vi "Process.vi"(8 "error in":errorcluster, 11 "Logger.syslog":refnum<class "Logger.syslog.lvclass">) -> (0 "error out":errorcluster, 3 "Logger.syslog out":refnum<class "Logger.syslog.lvclass">)   [LabVIEW 2019, in "Logger.syslog.lvlib" / "Logger.syslog.lvclass"]
doc: "---------------------------------------------------------------\nJKI State Machine Objects™\nhttp://jki.net/state-machine-objects/\nCopyright (C) 2005-2015, JKI <info@jki.net>\nALL RIGHTS RESERVED"
uses:
  Logger.syslog.lvclass
  <vilib>/NI/syslog/_subVIs/TypeDefs/syslog_message_cluster.ctl
  <vilib>/NI/syslog/_subVIs/TypeDefs/syslog_facility_codes.ctl
  <vilib>/NI/syslog/_subVIs/TypeDefs/syslog_severity_codes.ctl
  Typedefs/PrivateEvents--Logger.syslog.syslog message.ctl
  Logger.syslog.lvclass/Logger.syslog.ctl
  <userlib>/LevyLab/Logger/Logger/Logger.lvclass
  <vilib>/JKI/JKI SMO/smo.lvlibp/SMO/SMO.lvclass
  C:/Program Files (x86)/National Instruments/LabVIEW 2019/user.lib/LevyLab/Logger/Logger/Logger.lvclass
  C:/Program Files (x86)/National Instruments/LabVIEW 2019/vi.lib/JKI/JKI SMO/smo.lvlibp/SMO/SMO.lvclass
  <userlib>/LevyLab/Debug/Debug.lvlib
panel:
  # "For instructions on how to use the JKI State Machine Objects, examples and video tutorials, visit:\nhttp://jki.net/state-machine-objects/\n\nJKI State Machine Objects™\nhttp://jki.net/state-machine-objects/\nCopyright (C) 2005-2015, JKI <info@jki.net>\nALL RIGHTS RESERVED"
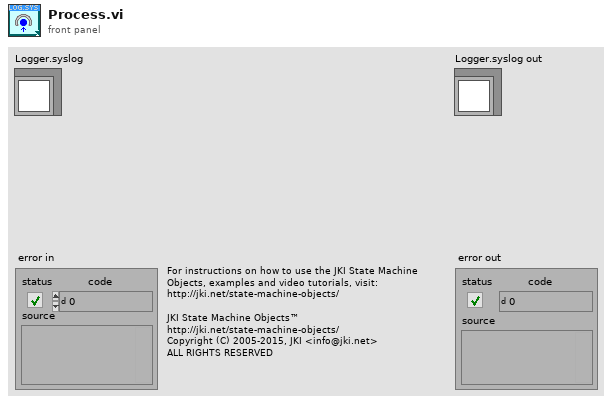
[diagram p1: front panel]
types:
  T1 = enum32{"invalid app kind", "Development System", "Run Time System", "Student Edition", "Embedded LabVIEW", "Evaluation", "Custom"}
  T2 = enum32{"Invalid", "Standard", "Closed", "Hidden", "Minimized", "Maximized"}
  T3 = enum16{"open", "replace", "create", "open or create", "replace or create", "replace or create with confirmation"}
  T4 = typedef "Logger.syslog.lvlib/Logger.syslog.lvclass/PrivateEvents--Logger.syslog.syslog message.ctl" = string
  T5 = typedef "syslog_message_cluster.ctl" = cluster{"Facility Code":T6, "Severity Code":T7, "Time Stamp":timestamp, "Hostname":string, "Message Tag":string, "Message Content":string}
  T6 = typedef "syslog_facility_codes.ctl" = enum16{"kernel", "user", "mail", "system daemons", "security/authorization", "syslogd", "line printer", "network news", "uucp", "clock daemon", "security/authorization (alternate)", "FTP daemon", "NTP subsystem", "log audit", "log alert", "clock daemon (alternate)", "local use 0", "local use 1", "local use 2", "local use 3", "local use 4", "local use 5", "local use 6", "local use 7"}
  T7 = typedef "syslog_severity_codes.ctl" = enum16{"emergency", "alert", "critical", "error", "warning", "notice", "info", "debug"}
  T8 = cluster{"Core":cluster{"Current VI Reference":refnum<vi>, "Close Panel on Exit?":bool, "Last Error":cluster{"error":errorcluster, "previous state":string, "remaining states":string}, "Shutdown?":bool}, "SelfRef":refnum<class "Logger.syslog.lvclass">, "collector port (514)":u16, "Syslog Collector Ref":refnum<k16>, "syslog message":T4, "Syslog Message":T5, "path":path}
  T9 = cluster{"Current VI Reference":refnum<vi>, "Close Panel on Exit?":bool, "Last Error":cluster{"error":errorcluster, "previous state":string, "remaining states":string}, "Shutdown?":bool}
  T10 = typedef "Debug.lvlib/Attribute.Debug.lvclass/DebugBehavior.ctl" = enum16{"Normal", "Debug"}
  T11 = typedef "smo.lvlibp/SMO.lvclass/Protected Events.ctl" = cluster{"StopProcesses":refnum<user-event>, "AbortProcesses":refnum<user-event>, "Config Changed":refnum<user-event>, "Dependency":refnum<user-event>}
  T12 = typedef "Logger.syslog.lvlib/Logger.syslog.lvclass/PrivateEvents--Cluster.ctl" = cluster{"syslog message":refnum<user-event>}
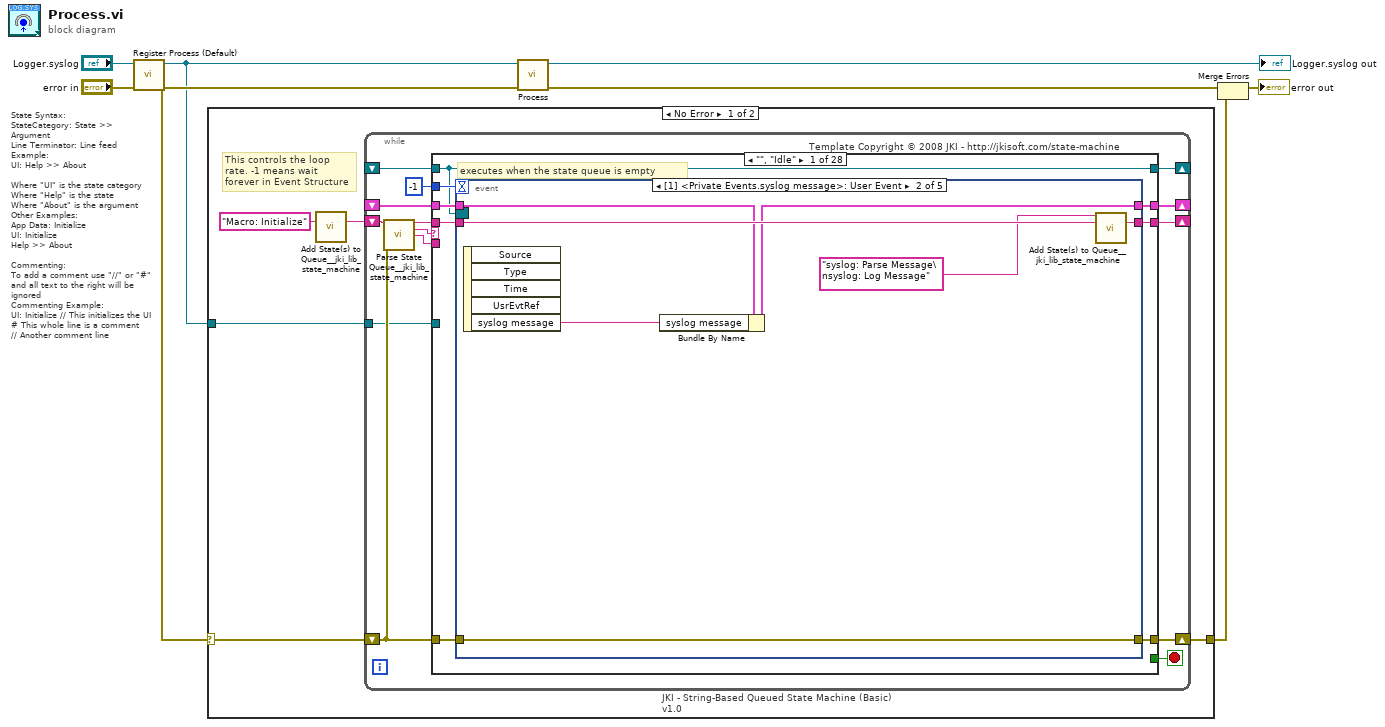
[diagram p0: block diagram]
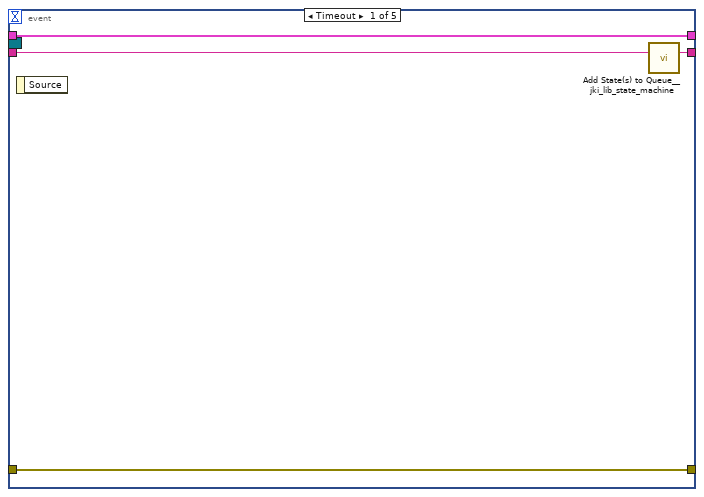
[diagram p2: hidden frame]
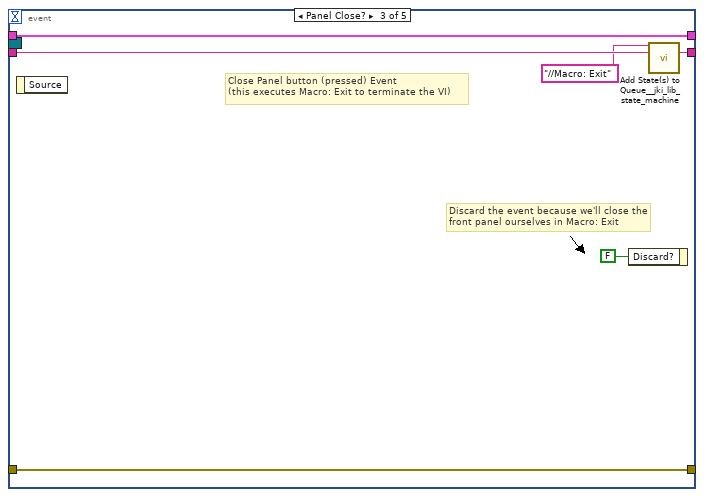
[diagram p3: hidden frame]
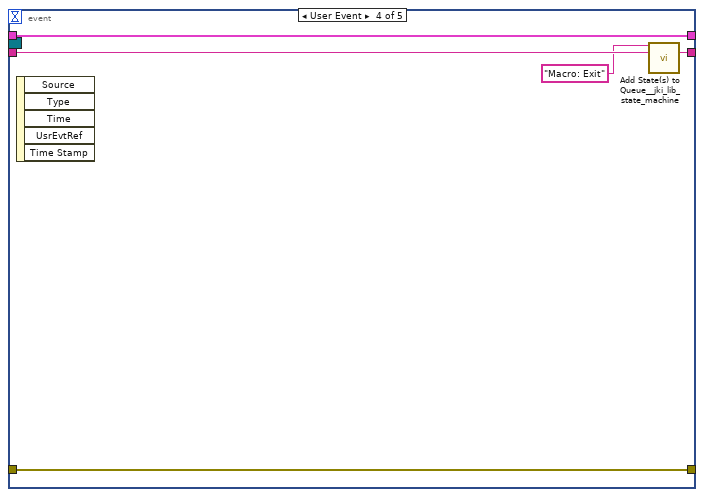
[diagram p4: hidden frame]
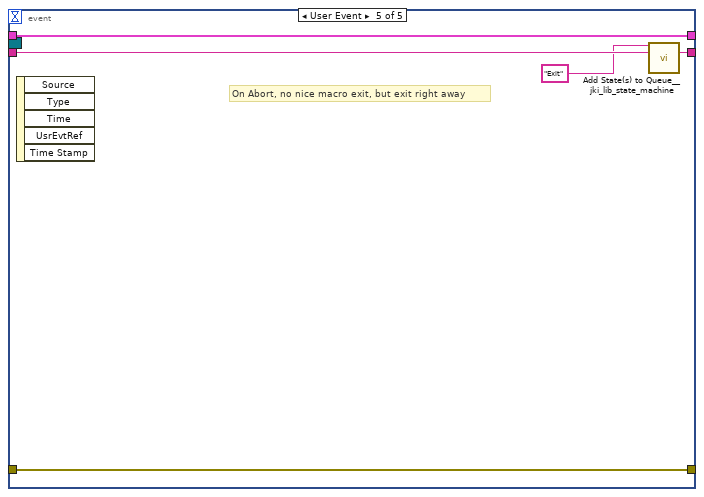
[diagram p5: hidden frame]
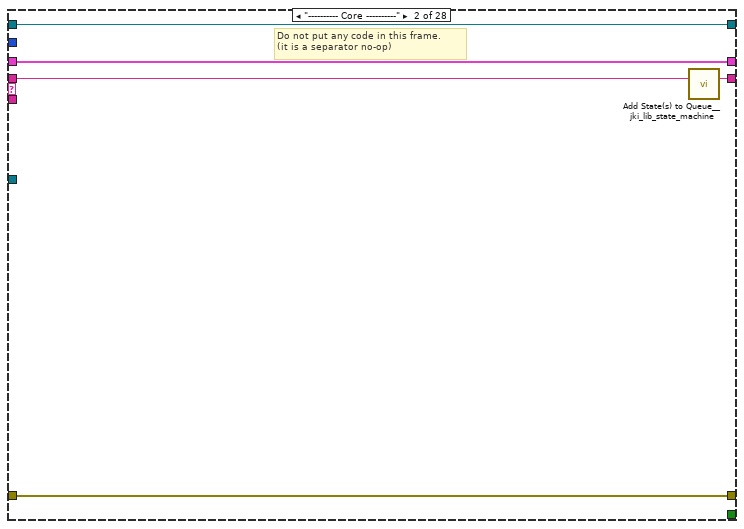
[diagram p6: hidden frame]
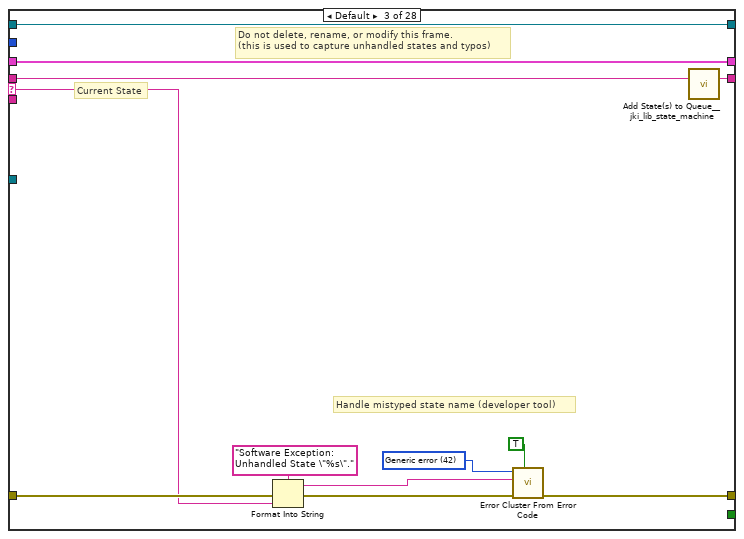
[diagram p7: hidden frame]
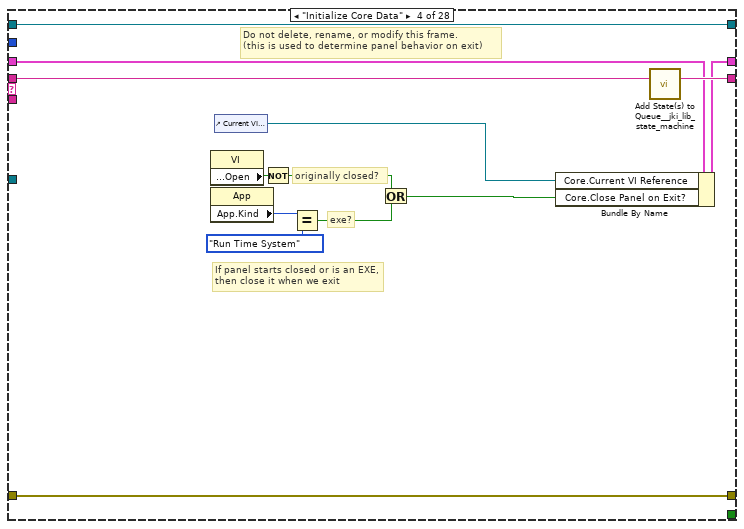
[diagram p8: hidden frame]
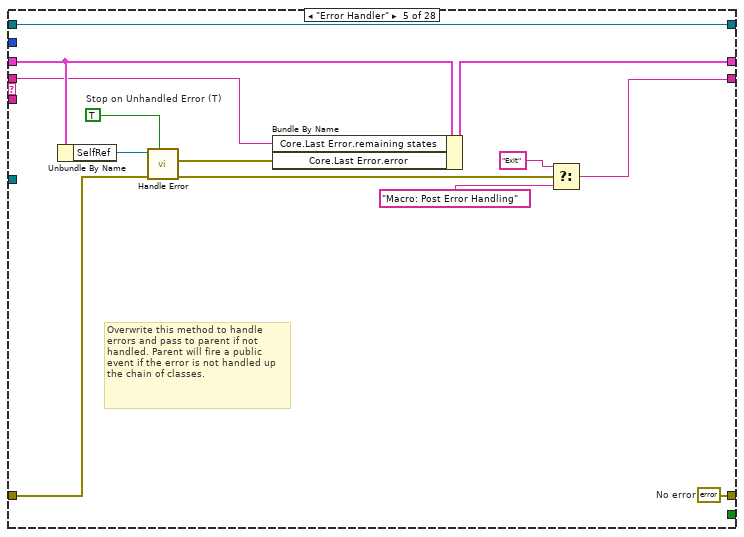
[diagram p9: hidden frame]
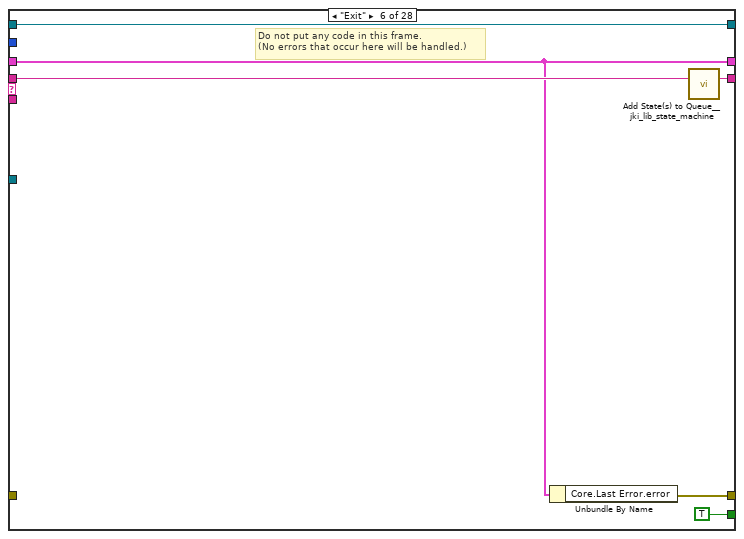
[diagram p10: hidden frame]
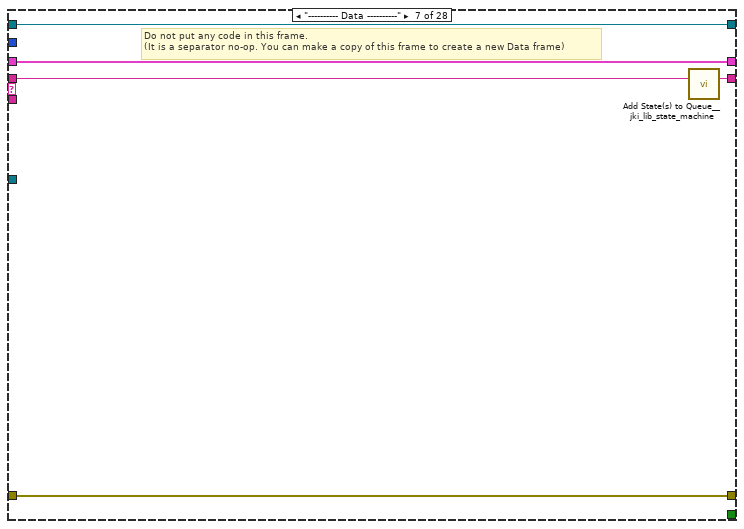
[diagram p11: hidden frame]
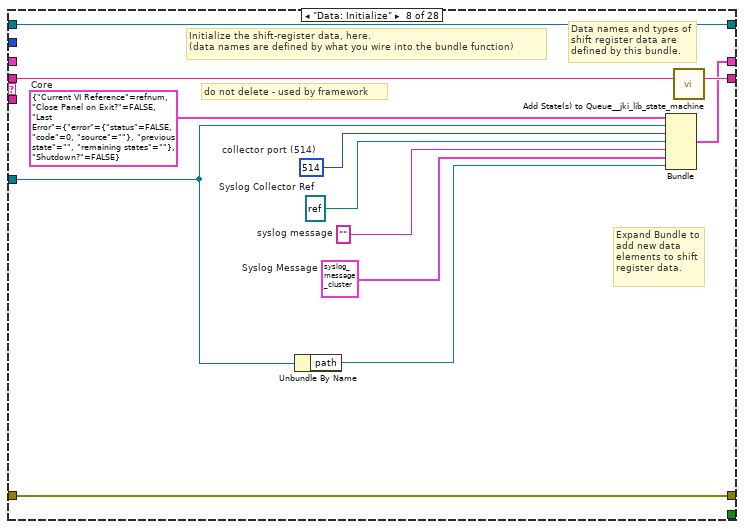
[diagram p12: hidden frame]
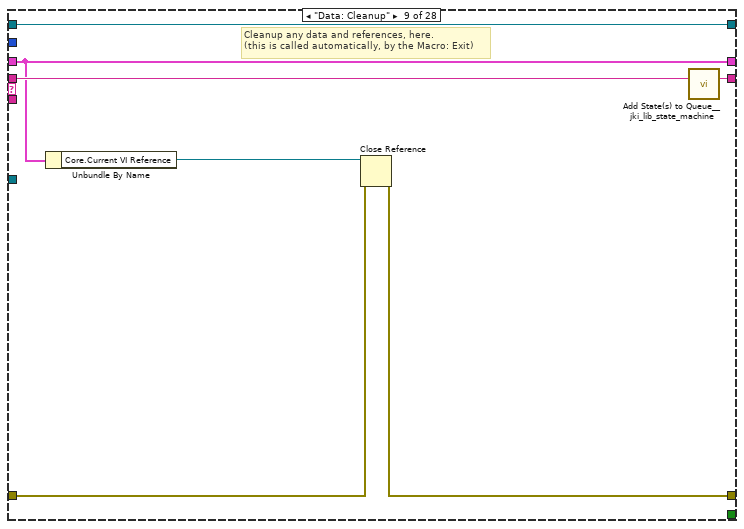
[diagram p13: hidden frame]
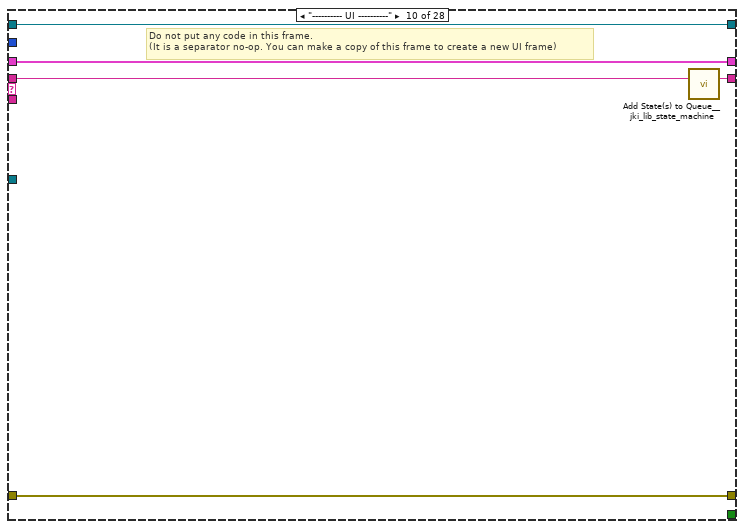
[diagram p14: hidden frame]
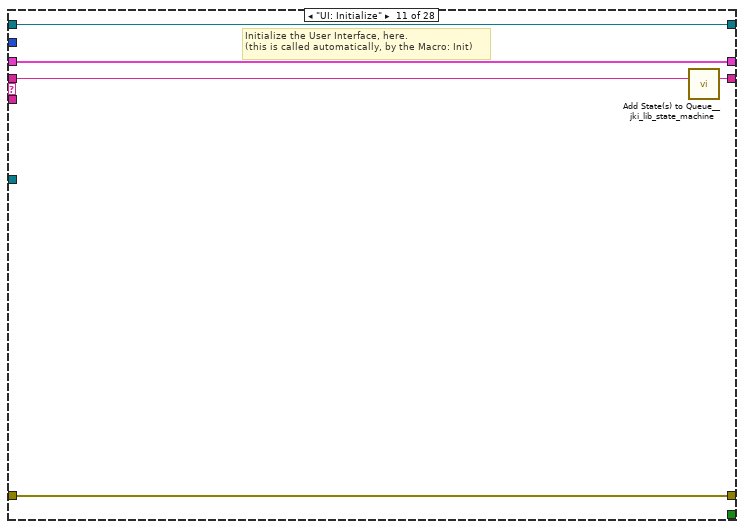
[diagram p15: hidden frame]
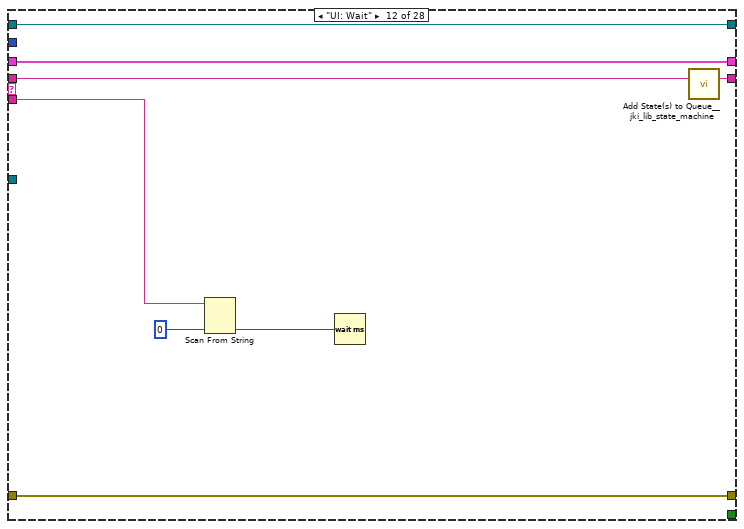
[diagram p16: hidden frame]
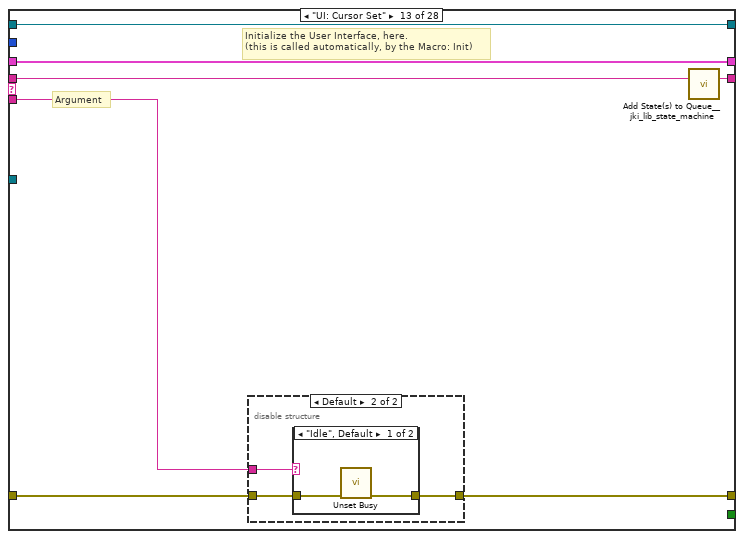
[diagram p17: hidden frame]
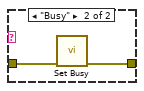
[diagram p19: hidden frame]
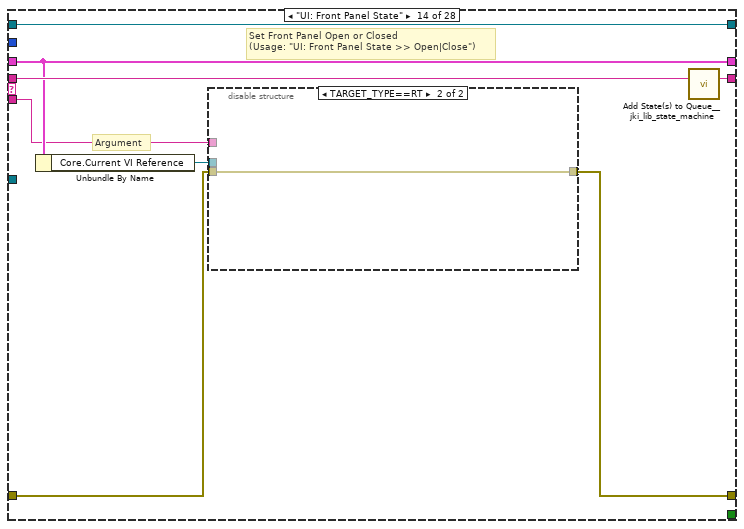
[diagram p20: hidden frame]
diagram:
  # "State Syntax:\nStateCategory: State >> Argument\nLine Terminator: Line feed\nExample:\nUI: Help >> About\n\nWhere \"UI\" is the state category\nWhere \"Help\" is the state\nWhere \"About\" is the argument\nOther Examples:\nApp Data: Initialize\nUI: Initialize\nHelp >> About\n\nCommenting:\nTo add a comment use \"//\" or \"#\" and all text to the right will be ignored\nCommenting Example:\nUI: Initialize // This initializes the UI\n# This whole line is a comment\n// Another comment line"
  n1 = call <vilib>:"Register Process (Default).vi"("error in (no error)"="error in", "SMO"="Logger.syslog") -> ("error out"=w5:errorcluster, "SelfRef"=w4:refnum<class "Logger.syslog.lvclass">)  [unwired: 8 in]
  n2 = case shown="No Error" w5 {
    selector: w5 -> [w10 w362]
    tunnel: w4 -> [w11 _]
    tunnel: [w9 w362] -> w1
    frame No Error {
      # "This controls the loop rate. -1 means wait forever in Event Structure"
      n3 = call <vilib>:"Add State(s) to Queue__jki_lib_state_machine.vi"("State(s) in (\"\")"="Macro: Initialize") -> ("States Out"=w13:string)  [unwired: 14 in]
      n4 = while "JKI - String-Based Queued State Machine (Basic) v1.0" {
        shift-right: [w20] -> _
        shift-left: _ -> [w19]
        shift-right: [w23] -> w9
        shift-left: w10 -> [w17]
        shift-right: [w22] -> _
        shift-left: w13 -> [w24]
        tunnel: w11 -> [w16]
        shift-right: [w15] -> _
        shift-left: _ -> [w14]
        stop <- w21 stop-if-true
        # "Template Copyright © 2008 JKI - http://jkisoft.com/state-machine"
        n5 = call <vilib>:"Parse State Queue__jki_lib_state_machine.vi"("State Queue"=w24, "Error In (no error)"=w17) -> ("Remaining States"=w26:string, "Current State"=w27:string, "Arguments"=w25:string)  [unwired: 11 in]
        n6 = case shown="\"\", \"Idle\"" w27 {
          selector: w27 -> [_ _ w69 _ _ _ _ _ _ _ _ _ _ _ _ _ _ _ _ _ _ _ _ _ _ _ _ _]
          tunnel: w26 -> [w35 w67 w73 w92 w93 w111 w116 w128 w135 w140 w145 w153 w160 w176 w208 w217 w232 w249 w269 w274 w285 w290 w303 w309 w314 w323 w331 w340]
          tunnel: w25 -> [_ _ _ _ _ _ _ _ _ _ _ w146 w154 w170 _ _ _ _ _ _ _ _ _ _ _ _ _ _]
          tunnel: w19 -> [w33 w64 w71 w83 w101 w107 w113 _ w130 w137 w143 w150 w158 w172 w205 w213 w221 w238 w255 w271 w282 w287 w301 w307 w312 w320 w325 w337]
          tunnel: [w32 w65 w75 w89 w102 w106 w114 w117 w131 w138 w142 w151 w155 w173 w206 w215 w219 w247 w267 w272 w276 w288 w296 w305 w310 w315 w328 w334] -> w23
          tunnel: w17 -> [w31 w65 w74 w89 w103 _ w114 w117 w132 w138 w142 w151 w156 w174 w206 w215 w218 w247 w267 w272 w277 w288 w297 w305 w310 w316 w328 w335]
          tunnel: [w34 w66 w72 w91 w95 w110 w115 w127 w134 w139 w144 w152 w159 w175 w207 w216 w231 w248 w268 w273 w284 w289 w302 w308 w313 w322 w330 w339] -> w22
          tunnel: [_ _ _ _ _ TRUE _ _ _ _ _ _ _ _ _ _ _ _ _ _ _ _ _ _ _ _ _ _] -> w21
          tunnel: [w30 w64 w71 w90 w100 w107 w113 w126 w130 w137 w143 w150 w158 w172 w205 w213 w222 w240 w256 w271 w282 w287 w301 w307 w312 w319 w326 w337] -> w20
          tunnel: -1 ("Timeout") -> [w29 _ _ _ _ _ _ _ _ _ _ _ _ _ _ _ _ _ _ _ _ _ _ _ _ _ _ _]
          tunnel: w16 -> [_ _ _ _ _ _ _ w118 _ _ _ _ _ _ _ _ _ _ _ _ _ _ _ _ _ _ _ _]
          tunnel: [w28 w63 w68 w80 w105 w108 w112 w125 w129 w136 w141 w149 w157 w169 w204 w214 w230 w246 w261 w270 w283 w286 w300 w306 w311 w321 w329 w338] -> w15
          tunnel: w14 -> [w28 w63 w68 w80 w105 w108 w112 w125 w129 w136 w141 w149 w157 w169 w204 w214 w230 w246 w261 w270 w283 w286 _ w306 w311 w321 w329 w338]
          frame "", "Idle" {
            # "executes when the state queue is empty"
            n7 = event shown="[1] <Private Events.syslog message>: User Event" {
              selector: w28 -> [_ _ _ _ _]
              dyn-events: _ -> [_ _ _ _ _]
              timeout: w29 -> [_ _ _ _ _]
              tunnel: w35 -> [w39 w46 w52 w57 w62]
              tunnel: [w38 w45 w51 w56 w61] -> w34
              tunnel: w33 -> [w37 w43 w49 w54 w59]
              tunnel: [w36 w44 w50 w55 w60] -> w32
              tunnel: w31 -> [w36 w44 w50 w55 w60]
              tunnel: [w37 w42 w49 w54 w59] -> w30
              event Timeout {
                n8 = event-data() -> ()  [unwired: 1 in, 1 out]
                n9 = call <vilib>:"Add State(s) to Queue__jki_lib_state_machine.vi"("State(s) in (\"\")"=w39) -> ("States Out"=w38:string)  [unwired: 14 in]
              }
              event User Event {
                n10 = event-data() -> ("syslog message"=w41:T4)  [unwired: 1 in, 4 out]
                n11 = Bundle By Name(cluster=w43, "syslog message"=w41) -> (w42:T8)
                n12 = call <vilib>:"Add State(s) to Queue__jki_lib_state_machine.vi"("State(s) in Front (\"\")"="syslog: Parse Message\nsyslog: Log Message" ("State(s) in Front (\"\")"), "State(s) in (\"\")"=w46) -> ("States Out"=w45:string)  [unwired: 13 in]
              }
              event Panel Close? {
                # "Discard the event because we'll close the front panel ourselves in Macro: Exit"
                # "Close Panel button (pressed) Event\n(this executes Macro: Exit to terminate the VI)"
                n13 = event-data() -> ()  [unwired: 1 in, 1 out]
                n14 = event-data("Discard?"=FALSE) -> ()  [unwired: 1 in, 1 out]
                n15 = call <vilib>:"Add State(s) to Queue__jki_lib_state_machine.vi"("State(s) in Front (\"\")"="//Macro: Exit", "State(s) in (\"\")"=w52) -> ("States Out"=w51:string)  [unwired: 13 in]
              }
              event User Event {
                n16 = event-data() -> ()  [unwired: 1 in, 5 out]
                n17 = call <vilib>:"Add State(s) to Queue__jki_lib_state_machine.vi"("State(s) in Front (\"\")"="Macro: Exit", "State(s) in (\"\")"=w57) -> ("States Out"=w56:string)  [unwired: 13 in]
              }
              event User Event {
                # "On Abort, no nice macro exit, but exit right away"
                n18 = event-data() -> ()  [unwired: 1 in, 5 out]
                n19 = call <vilib>:"Add State(s) to Queue__jki_lib_state_machine.vi"("State(s) in Front (\"\")"="Exit", "State(s) in (\"\")"=w62) -> ("States Out"=w61:string)  [unwired: 13 in]
              }
            }
          }
          frame "---------- Core ----------" {
            # "Do not put any code in this frame.\n(it is a separator no-op)"
            n20 = call <vilib>:"Add State(s) to Queue__jki_lib_state_machine.vi"("State(s) in (\"\")"=w67) -> ("States Out"=w66:string)  [unwired: 14 in]
          }
          frame Default {
            w78 = 42 items=["No error", "Argument error", "Memory is full", "Out of zone", "End of file", "File already open", "Generic file I/O error", "File not found", "File permission error", "Disk is full", "Duplicate path", "Too many files open", "System feature not enabled", "Resource file not found", "Cannot add resource", "Resource not found", "Image not found", "Image memory error", "Pen does not exist", "Config type invalid", "Config token not found", "Config parse error", "Config memory error", "Bad external code format", "Bad external code offset", "External code not present", "Null window", "Destroy window error", "Null menu", "Print aborted", "Bad print record", "Print driver error", "Windows error during printing", "Memory error during printing", "Print dialog error", "Generic print error", "Invalid device refnum", "Device not found", "Device parameter error", "Device unit error", "Cannot open device", "Device call aborted", "Generic error", "Cancelled by user", "Object ID too low", "Object ID too high", "Object not in heap", "Unknown heap", "Unknown object (invalid DefProc)", "Unknown object (DefProc not in table)", "Message out of range", "Invalid (null) method", "Unknown message", "Manager call not supported", "Bad address", "Network operation in progress", "Network operation timed out", "Connection is busy", "Network attribute not supported", "Network error", "Address in use", "System out of memory", "Connection aborted", "Connection refused", "Not connected", "Already connected", "Connection closed", "Initialization error (interapplication manager)", "Bad occurrence", "Wait on unbound occurrence handler", "Occurrence queue overflow", "Datalog type conflict", "Unused", "Unrecognized type (interapplication manager)", "Memory corrupt", "Failed to make temporary DLL", "Old CIN version", "Drag socket not found", "Failed to load drop-object", "Failed to register OLE object", "Failed to release OLE object", "Format specifier type mismatch", "Unknown format specifier", "Too few format specifiers", "Too many format specifiers", "Scan failed", "Newer CIN version", "Error converting to variant", "Runtime menu error", "Password tampered", "Variant attribute not found", "Incompatible variant data type", "Event data is not available", "Event Store is not present", "Occurrence is not found", "Event Queue is not created", "Event info is not available", "Refnum passed is NULL", "Error retrieving Class GUID", "Error retrieving CoClass GUID", "Error retrieving TypeLib GUID.", "Bad built application magic bytes.", "Specific driver is different from the specific driver associated with the Logical Name.", "There is no session opened to the class driver.", "Max Error", "MAX - Error with config objects", "MAX - Error loading configuration", "MAX - Group not supported"]
            # "Current State"
            # "Do not delete, rename, or modify this frame.\n(this is used to capture unhandled states and typos)"
            # "Handle mistyped state name (developer tool)"
            n21 = Format Into String(format string="Software Exception: Unhandled State \"%s\"." ("message"), error in=w74, w69) -> (resulting string=w77:string, error out=w76:errorcluster)  [unwired: 1 in]
            n22 = call <vilib>:"Error Cluster From Error Code.vi"("show call chain? (False)"=TRUE, "error in (no error)"=w76, "error message (\"\")"=w77, "error code (0)"=w78) -> ("error out"=w75:errorcluster)  [unwired: 5 in]
            n23 = call <vilib>:"Add State(s) to Queue__jki_lib_state_machine.vi"("State(s) in (\"\")"=w73) -> ("States Out"=w72:string)  [unwired: 14 in]
          }
          frame "Initialize Core Data" {
            # "Do not delete, rename, or modify this frame.\n(this is used to determine panel behavior on exit)"
            # "originally closed?"
            # "exe?"
            # "If panel starts closed or is an EXE, then close it when we exit"
            n24 = property class="VI"() -> ("Front Panel.Open"=w88:bool)  [unwired: 2 in, 2 out]
            n25 = property class="App"() -> ("App.Kind"=w87:T1)  [unwired: 2 in, 2 out]
            n26 = control-ref of="Current VI Reference"() -> (w81:refnum<vi>)
            n27 = Not(x=w88) -> (.not. x?=w85:bool)
            n28 = Equal?(x=w87, y=T1."Run Time System" ("Application:Kind")) -> (x = y?=w84:bool)
            n29 = Or(x=w85, y=w84) -> (x .or. y?=w82:bool)
            n30 = Bundle By Name(cluster=w83, "Core.Current VI Reference"=w81, "Core.Close Panel on Exit?"=w82) -> (w90:T8)
            n31 = call <vilib>:"Add State(s) to Queue__jki_lib_state_machine.vi"("State(s) in (\"\")"=w92) -> ("States Out"=w91:string)  [unwired: 14 in]
          }
          frame "Error Handler" {
            w96 = TRUE  # Stop on Unhandled Error (T)
            w102 = errorcluster {"status"=FALSE, "code"=0, "source"=""}  # No error
            # "Overwrite this method to handle errors and pass to parent if not handled. Parent will fire a public event if the error is not handled up the chain of classes."
            n32 = Unbundle By Name(w101) -> ("SelfRef"=w104:refnum<class "Logger.syslog.lvclass">)
            n33 = call-dynamic "Handle Error.vi"("Stop on Unhandled Error (T)"=w96, "error in"=w103, "SMO"=w104) -> ("handling error"=w97:errorcluster, "Unhandled error"=w99:errorcluster)  [unwired: 6 in, 1 out]
            n34 = Bundle By Name(cluster=w101, "Core.Last Error.remaining states"=w93, "Core.Last Error.error"=w99) -> (w100:T8)
            n35 = Select(t="Exit", s=w97, f="Macro: Post Error Handling") -> (s? t:f=w95:string)
          }
          frame "Exit" {
            # "Do not put any code in this frame.\n(No errors that occur here will be handled.)"
            n36 = Unbundle By Name(w107) -> ("Core.Last Error.error"=w106:errorcluster)
            n37 = call <vilib>:"Add State(s) to Queue__jki_lib_state_machine.vi"("State(s) in (\"\")"=w111) -> ("States Out"=w110:string)  [unwired: 14 in]
          }
          frame "---------- Data ----------" {
            # "Do not put any code in this frame.\n(It is a separator no-op. You can make a copy of this frame to create a new Data frame)"
            n38 = call <vilib>:"Add State(s) to Queue__jki_lib_state_machine.vi"("State(s) in (\"\")"=w116) -> ("States Out"=w115:string)  [unwired: 14 in]
          }
          frame "Data: Initialize" {
            w121 = T4 ""  # syslog message
            w120 = T5 {"Facility Code"=enum."kernel", "Severity Code"=enum."emergency", "Time Stamp"=timestamp(0 s since 1904-01-01), "Hostname"="", "Message Tag"="", "Message Content"=""}  # Syslog Message
            w122 = refnum<k16> refnum  # Syslog Collector Ref
            w123 = u16 514  # collector port (514)
            w124 = T9 {"Current VI Reference"=refnum, "Close Panel on Exit?"=FALSE, "Last Error"={"error"={"status"=FALSE, "code"=0, "source"=""}, "previous state"="", "remaining states"=""}, "Shutdown?"=FALSE}  # Core
            # "do not delete - used by framework"
            # "Expand Bundle to add new data elements to shift register data."
            # "Data names and types of shift register data are defined by this bundle."
            # "Initialize the shift-register data, here.\n(data names are defined by what you wire into the bundle function)"
            n39 = Unbundle By Name(w118) -> ("path"=w119:path)
            n40 = Bundle("Core"=w124, "SelfRef"=w118, "collector port (514)"=w123, "Syslog Collector Ref"=w122, "syslog message"=w121, "Syslog Message"=w120, "path"=w119) -> (w126:T8)  [unwired: 1 in]
            n41 = call <vilib>:"Add State(s) to Queue__jki_lib_state_machine.vi"("State(s) in (\"\")"=w128) -> ("States Out"=w127:string)  [unwired: 14 in]
          }
          frame "Data: Cleanup" {
            # "Cleanup any data and references, here.\n(this is called automatically, by the Macro: Exit)"
            n42 = Unbundle By Name(w130) -> ("Core.Current VI Reference"=w133:refnum<vi>)
            n43 = Close Reference(reference=w133, error in (no error)=w132) -> (error out=w131:errorcluster)
            n44 = call <vilib>:"Add State(s) to Queue__jki_lib_state_machine.vi"("State(s) in (\"\")"=w135) -> ("States Out"=w134:string)  [unwired: 14 in]
          }
          frame "---------- UI ----------" {
            # "Do not put any code in this frame.\n(It is a separator no-op. You can make a copy of this frame to create a new UI frame)"
            n45 = call <vilib>:"Add State(s) to Queue__jki_lib_state_machine.vi"("State(s) in (\"\")"=w140) -> ("States Out"=w139:string)  [unwired: 14 in]
          }
          frame "UI: Initialize" {
            # "Initialize the User Interface, here.\n(this is called automatically, by the Macro: Init)"
            n46 = call <vilib>:"Add State(s) to Queue__jki_lib_state_machine.vi"("State(s) in (\"\")"=w145) -> ("States Out"=w144:string)  [unwired: 14 in]
          }
          frame "UI: Wait" {
            n47 = Scan From String(input string=w146, default 1=u32 0) -> (output 1=w147:u32)  [unwired: 3 in, 3 out]
            n48 = Wait (ms)(milliseconds to wait=w147) -> ()  [unwired: 1 out]
            n49 = call <vilib>:"Add State(s) to Queue__jki_lib_state_machine.vi"("State(s) in (\"\")"=w153) -> ("States Out"=w152:string)  [unwired: 14 in]
          }
          frame "UI: Cursor Set" {
            # "Argument"
            # "Initialize the User Interface, here.\n(this is called automatically, by the Macro: Init)"
            n50 = disable-structure shown="Default" {
              disable-tunnel: w156 -> [w161 w164]
              disable-tunnel: [w161 w163] -> w155
              disable-tunnel: w154 -> [_ w162]
              frame condition #0 {
              }
              frame condition #1 (active) {
                n51 = case shown="\"Idle\", Default" w162 {
                  tunnel: w164 -> [w166 w168]
                  tunnel: [w165 w167] -> w163
                  frame "Idle", Default {
                    n52 = call <vilib>:"Unset Busy.vi"("error in (no error)"=w166) -> ("error out"=w165:errorcluster)  [unwired: 10 in]
                  }
                  frame "Busy" {
                    n53 = call <vilib>:"Set Busy.vi"("error in (no error)"=w168) -> ("error out"=w167:errorcluster)  [unwired: 9 in, 1 out]
                  }
                }
              }
            }
            n54 = call <vilib>:"Add State(s) to Queue__jki_lib_state_machine.vi"("State(s) in (\"\")"=w160) -> ("States Out"=w159:string)  [unwired: 14 in]
          }
          frame "UI: Front Panel State" {
            # "Argument"
            # "Set Front Panel Open or Closed\n(Usage: \"UI: Front Panel State >> Open|Close\")"
            n55 = Unbundle By Name(w172) -> ("Core.Current VI Reference"=w171:refnum<vi>)
            n56 = disable-structure shown="TARGET_TYPE==RT" {
              disable-tunnel: w174 -> [w180 w203]
              disable-tunnel: [w179 w203] -> w173
              disable-tunnel: w171 -> [w178 _]
              disable-tunnel: w170 -> [w177 _]
              frame condition #0 (active) {
                n57 = case shown="\"Close\"" w177 {
                  tunnel: w180 -> [w184 w197]
                  tunnel: [w186 w198] -> w179
                  tunnel: w178 -> [w185 w195]
                  frame "Open", Default {
                    n58 = property class="VI"(reference=w185, error in=w184) -> (reference out=w182:refnum<vi>, error out=w183:errorcluster, "FP.State"=w181:T2)
                    n59 = case shown="\"Closed\"" w181 {
                      tunnel: [w189 w192] -> w186
                      tunnel: w183 -> [w188 w192]
                      tunnel: w182 -> [w187 _]
                      frame "Closed" {
                        n60 = invoke class="VI" method="FP.Open"(reference=w187, error in=w188, "Activate"=TRUE, "State"=T2."Standard") -> (error out=w189:errorcluster)  [unwired: 1 in, 4 out]
                      }
                      frame Default {
                      }
                    }
                  }
                  frame "Close" {
                    n61 = property class="VI"(reference=w195, error in=w197) -> (reference out=w194:refnum<vi>, error out=w196:errorcluster, "FP.State"=w193:T2)
                    n62 = case shown="Default" w193 {
                      tunnel: [w199 w202] -> w198
                      tunnel: w196 -> [w199 w201]
                      tunnel: w194 -> [_ w200]
                      frame "Invalid", "Closed" {
                      }
                      frame Default {
                        n63 = invoke class="VI" method="FP.Close"(reference=w200, error in=w201) -> (error out=w202:errorcluster)  [unwired: 1 in, 2 out]
                      }
                    }
                  }
                }
              }
              frame condition #1 {
              }
            }
            n64 = call <vilib>:"Add State(s) to Queue__jki_lib_state_machine.vi"("State(s) in (\"\")"=w176) -> ("States Out"=w175:string)  [unwired: 14 in]
          }
          frame "---------- Macro ----------" {
            # "Do not put any code in this frame.\n(It is a separator no-op. You can make a copy of this frame to create a new Macro frame)"
            n65 = call <vilib>:"Add State(s) to Queue__jki_lib_state_machine.vi"("State(s) in (\"\")"=w208) -> ("States Out"=w207:string)  [unwired: 14 in]
          }
          frame "Macro: Initialize" {
            w211 = "UI: Initialize\nUI: Front Panel State >> Close\nMacro: Debug"  # UI: Initialize UI: Front Panel State >> Close Macro: Debug
            # "Initialization Macro\n(This is called once, when the VI starts)"
            n66 = call <vilib>:"Add State(s) to Queue__jki_lib_state_machine.vi"("State(s) in Front (\"\")"="Data: Initialize\nInitialize Core Data\nEvents: Register", "State(s) in (\"\")"="Process: Sync", "State(s) at Back (\"\")"=w211) -> ("States Out"=w210:string)  [unwired: 12 in]
            n67 = call <vilib>:"Add State(s) to Queue__jki_lib_state_machine.vi"("State(s) in Front (\"\")"=w210, "State(s) in (\"\")"=w217) -> ("States Out"=w216:string)  [unwired: 13 in]
          }
          frame "Macro: Debug" {
            # "Macro: Debug\n(get debug behavior, determine UI and determine shutdown behavior)"
            # "exe?"
            # "If pane is an EXE, then close it when we exit"
            n68 = Unbundle By Name(w221) -> ("Core.Close Panel on Exit?"=w224:bool, "SelfRef"=w229:refnum<class "Logger.syslog.lvclass">)
            n69 = property class="App"() -> ("App.Kind"=w227:T1)  [unwired: 2 in, 2 out]
            n70 = Equal?(x=w227, y=T1."Run Time System" ("Application:Kind")) -> (x = y?=w223:bool)
            n71 = call <userlib>:"Get Debug Mode.vi"("error in (no error)"=w218, "SMO"=w229) -> ("error out"=w219:errorcluster, "Behavior"=w228:T10)  [unwired: 7 in, 1 out]
            n72 = case shown="\"Debug\"" w228 {
              tunnel: [_ "UI: Front Panel State >> Open\nUI: Wait >> 1000"] -> w220
              tunnel: [w233 w234] -> w225
              tunnel: w224 -> [w233 _]
              tunnel: w223 -> [_ w236]
              frame "Normal", Default {
                # "respect core.close"
              }
              frame "Debug" {
                # "keep panel open\nunless exe"
                n73 = Or(x=w236, y=FALSE) -> (x .or. y?=w234:bool)
              }
            }
            n74 = Bundle By Name(cluster=w221, "Core.Close Panel on Exit?"=w225) -> (w222:T8)
            n75 = call <vilib>:"Add State(s) to Queue__jki_lib_state_machine.vi"("State(s) in Front (\"\")"=w220, "State(s) in (\"\")"=w232) -> ("States Out"=w231:string)  [unwired: 13 in]
          }
          frame "Macro: Post Error Handling" {
            # "Clear Last Error?"
            n76 = Unbundle By Name(w238) -> ("Core.Last Error.remaining states"=w241:string, "Core.Shutdown?"=w242:bool)
            n77 = Unbundle By Name(w238) -> ("Core.Last Error.error"=w245:errorcluster)
            n78 = case shown="False" FALSE {
              tunnel: w245 -> [w253 _]
              tunnel: [w253 _] -> w244
              frame False {
              }
              frame True {
              }
            }
            n79 = case shown="True" w242 {
              tunnel: w241 -> [w250 w252]
              tunnel: [w250 w251] -> w239
              frame False {
                # "These are the remaining states (at the moment the error occured). States can be altered according to business logic."
                # "NOT SHUTTING DOWN"
              }
              frame True {
                # "Developer can decide to alter the states but should be aware that during the shutdown process, there are certain states that must be run for the SMO to properly shut itself (and this process) down. As such, one can add states to perform additional clean-ups, but should append the remaining state to be executed."
                # "SHUTTING DOWN"
                n80 = call <vilib>:"Add State(s) to Queue__jki_lib_state_machine.vi"("State(s) in (\"\")"=w252) -> ("States Out"=w251:string)  [unwired: 14 in]
              }
            }
            n81 = Bundle By Name(cluster=w238, "Core.Last Error.error"=w244) -> (w240:T8)
            n82 = call <vilib>:"Add State(s) to Queue__jki_lib_state_machine.vi"("State(s) in Front (\"\")"=w239, "State(s) in (\"\")"=w249) -> ("States Out"=w248:string)  [unwired: 13 in]
          }
          frame "Macro: Exit" {
            # "Exit Macro\n(This is called once, when the VI exits)"
            n83 = Unbundle By Name(w255) -> ("Core.Close Panel on Exit?"=w266:bool)
            n84 = Bundle By Name(cluster=w255, "Core.Shutdown?"=TRUE) -> (w256:T8)
            n85 = Select(t="UI: Front Panel State >> Close", s=w266, f="") -> (s? t:f=w263:string)
            n86 = call <vilib>:"Add State(s) to Queue__jki_lib_state_machine.vi"("State(s) in Front (\"\")"="Data: Cleanup\nEvents: Unregister", "State(s) in (\"\")"="Process: Sync", "State(s) at Back (\"\")"="Exit") -> ("States Out"=w258:string)  [unwired: 12 in]
            n87 = call <vilib>:"Add State(s) to Queue__jki_lib_state_machine.vi"("State(s) in (\"\")"=w263, "State(s) at Back (\"\")"=w258) -> ("States Out"=w262:string)  [unwired: 13 in]
            n88 = call <vilib>:"Add State(s) to Queue__jki_lib_state_machine.vi"("State(s) in Front (\"\")"=w262, "State(s) in (\"\")"=w269) -> ("States Out"=w268:string)  [unwired: 13 in]
          }
          frame "---------- Process ----------" {
            # "Template Separator\n(You can make a copy of, or modify, this frame)"
            n89 = call <vilib>:"Add State(s) to Queue__jki_lib_state_machine.vi"("State(s) in (\"\")"=w274) -> ("States Out"=w273:string)  [unwired: 14 in]
          }
          frame "Process: Sync" {
            n90 = Unbundle By Name(w282) -> ("SelfRef"=w278:refnum<class "Logger.syslog.lvclass">)
            n91 = call <vilib>:"WaitOnProcessSync.vi"("error in (no error)"=w277, "SMO"=w278) -> ("error out"=w276:errorcluster, "Don't run?"=w281:bool)  [unwired: 7 in, 1 out]
            n92 = Select(t="Data: Cleanup\nEvents: Unregister\nExit", s=w281, f="") -> (s? t:f=w275:string)
            n93 = call <vilib>:"Add State(s) to Queue__jki_lib_state_machine.vi"("State(s) in Front (\"\")"=w275, "State(s) in (\"\")"=w285) -> ("States Out"=w284:string)  [unwired: 13 in]
          }
          frame "---------- Events ----------" {
            # "Template Separator\n(You can make a copy of, or modify, this frame)"
            n94 = call <vilib>:"Add State(s) to Queue__jki_lib_state_machine.vi"("State(s) in (\"\")"=w290) -> ("States Out"=w289:string)  [unwired: 14 in]
          }
          frame "Events: Register" {
            # "Expand to add\nmore events"
            n95 = Unbundle By Name(w301) -> ("SelfRef"=w298:refnum<class "Logger.syslog.lvclass">)
            n96 = call <vilib>:"GetProtectedEvents.vi"("SMO"=w298) -> ("error out"=w294:errorcluster, "SMO Protected Events"=w299:T11, "SMO out"=w293:refnum<class "Logger.syslog.lvclass">)  [unwired: 8 in]
            n97 = call "Logger.syslog.GetPrivateEvents.vi"("Logger.syslog"=w293) -> ("error out"=w291:errorcluster, "Private Events"=w292:T12)  [unwired: 8 in, 1 out]
            n98 = register-events(w299, w292) -> (reference out=w300:refnum<event-registration>, error out=w295:errorcluster)  [unwired: 2 in]
            n99 = Merge Errors(w291, w297, w295, w294) -> (w296:errorcluster)
            n100 = call <vilib>:"Add State(s) to Queue__jki_lib_state_machine.vi"("State(s) in (\"\")"=w303) -> ("States Out"=w302:string)  [unwired: 14 in]
          }
          frame "Events: Unregister" {
            n101 = Unregister For Events(event registration refnum=w306, error in=w305) -> (error out=w304:errorcluster)
            n102 = call <vilib>:"Clear Errors.vi"("error in (no error)"=w304) -> ()  [unwired: 5 in, 2 out]
            n103 = call <vilib>:"Add State(s) to Queue__jki_lib_state_machine.vi"("State(s) in (\"\")"=w309) -> ("States Out"=w308:string)  [unwired: 14 in]
          }
          frame "---------- syslog ----------" {
            n104 = call <vilib>:"Add State(s) to Queue__jki_lib_state_machine.vi"("State(s) in (\"\")"=w314) -> ("States Out"=w313:string)  [unwired: 14 in]
          }
          frame "syslog: Start UDP Collector" {
            n105 = Unbundle By Name(w320) -> ("collector port (514)"=w318:u16)
            n106 = call <vilib>:"Syslog Collector Init.vi"("error in (no error)"=w316, "collector port (514)"=w318) -> ("error out"=w315:errorcluster, "Syslog Collector Ref"=w317:refnum<k16>)  [unwired: 8 in]
            n107 = Bundle By Name(cluster=w320, "Syslog Collector Ref"=w317) -> (w319:T8)
            n108 = call <vilib>:"Add State(s) to Queue__jki_lib_state_machine.vi"("State(s) in (\"\")"=w323) -> ("States Out"=w322:string)  [unwired: 14 in]
          }
          frame "syslog: Parse Message" {
            n109 = Unbundle By Name(w325) -> ("syslog message"=w324:T4)
            n110 = call <vilib>:"syslog_Message Parse.vi"("syslog message"=w324) -> ("Syslog Message"=w327:T5)  [unwired: 10 in]
            n111 = Bundle By Name(cluster=w325, "Syslog Message"=w327) -> (w326:T8)
            n112 = call <vilib>:"Add State(s) to Queue__jki_lib_state_machine.vi"("State(s) in (\"\")"=w331) -> ("States Out"=w330:string)  [unwired: 14 in]
          }
          frame "syslog: Log Message" {
            n113 = Unbundle By Name(w337) -> ("path"=w332:path, "syslog message"=w336:T4)
            n114 = case shown="No Error" w335 {
              selector: w335 -> [w342 w356]
              tunnel: w336 -> [w352 _]
              tunnel: [w343 w358] -> w334
              tunnel: "local" ("syslog client address") -> [w353 _]
              tunnel: w332 -> [w341 _]
              frame No Error {
                n115 = Format Into String(format string="%s: %s\\r\\n" ("string"), w353, w352) -> (resulting string=w355:string)  [unwired: 2 in, 1 out]
                n116 = Open/Create/Replace File(file path (use dialog)=w341, error in=w342, operation (0:open)=T3."open or create") -> (refnum out=w348:refnum<file>, error out=w349:errorcluster)  [unwired: 3 in, 1 out]
                n117 = Set File Position(refnum=w348, from (0:start)=enum16{"start", "end", "current"}."end", error in=w349) -> (refnum out=w347:refnum<file>, error out=w350:errorcluster)  [unwired: 1 in]
                n118 = Write to Text File(file (use dialog)=w347, text=w355, error in=w350) -> (refnum out=w345:refnum<file>, error out=w344:errorcluster)  [unwired: 1 in, 1 out]
                n119 = Close File(refnum=w345, error in=w344) -> (error out=w343:errorcluster)  [unwired: 1 out]
              }
              frame Error {
                n120 = Unbundle By Name(w356) -> ("code"=w357:i32)
                n121 = case shown="56" w357 {
                  tunnel: w356 -> [w360 w361]
                  tunnel: [w359 w361] -> w358
                  frame 56 {
                    # "Clear the Timeout error"
                    n122 = call <vilib>:"Clear Errors.vi"("error in (no error)"=w360) -> ("error out"=w359:errorcluster)  [unwired: 5 in, 1 out]
                  }
                  frame Default {
                  }
                }
              }
            }
            n123 = call <vilib>:"Add State(s) to Queue__jki_lib_state_machine.vi"("State(s) in (\"\")"=w340) -> ("States Out"=w339:string)  [unwired: 14 in]
          }
        }
      }
    }
    frame Error {
    }
  }
  n124 = call-parent "Process.vi"("error in"=w5, "Logger"=w4) -> ("error out"=w2:errorcluster, "Logger out"=→"Logger.syslog out":refnum<class "Logger.syslog.lvclass">)  [unwired: 8 in]
  n125 = Merge Errors(w2, w1) -> (→"error out":errorcluster)
